vi "Motor Status Wait Z.vi"(2 "Error In":errorcluster, 3 "Reference In":refnum<class "_Controller.lvclass">) -> (0 "Error Out":errorcluster, 1 "Reference Out":refnum<class "_Controller.lvclass">)   [LabVIEW 2020]
doc: "Waits for motor Z to be in idle (i.e. not moving). This is done to ensure motor Z has completed any neccessary movement before sending the next command. Otherwise a pulsing error is obtained.\n\nArgs:\n\nReference In: Incoming communication (reference) between LabView and the scanning rig controller\nError In: Checks for any errors with the incoming communication (reference)\n\nReturns:\n\nReference Out: Output communnication (reference) between LabView and controller\nError Out: Checks for any error with output communication (reference)"
uses:
  <instrlib>/Arcus Ethernet Driver 1.0.0/ArcusEthernetComm/classes/Controller/_Controller.lvclass
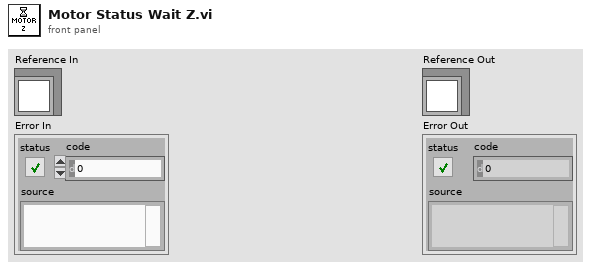
[diagram p1: front panel]
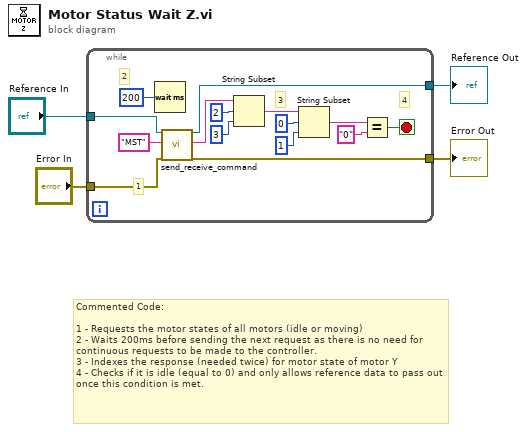
[diagram p0: block diagram]
diagram:
  # "Commented Code:\n\n1 - Requests the motor states of all motors (idle or moving)\n2 - Waits 200ms before sending the next request as there is no need for continuous requests to be made to the controller. \n3 - Indexes the response (needed twice) for motor state of motor Y\n4 - Checks if it is idle (equal to 0) and only allows reference data to pass out once this condition is met."
  n1 = while {
    tunnel: "Reference In" -> [w14]
    tunnel: "Error In" -> [w13]
    tunnel: [w10] -> w2
    tunnel: [w9] -> w1
    stop <- w11 stop-if-true
    # "4"
    # "3"
    # "2"
    # "1"
    n2 = Wait (ms)(milliseconds to wait=u32 200) -> ()  [unwired: 1 out]
    n3 = call <instrlib>:"send_receive_command.vi"("reference (in)"=w14, "ASCII Command (in)"="MST", "error in (no error)"=w13) -> ("reference (out)"=w10:refnum<class "_Controller.lvclass">, "response (out)"=w15:string, "error out"=w9:errorcluster)  [unwired: 12 in, 2 out]
    n4 = String Subset(string=w15, offset (0)=2, length (rest)=3 ("length (rest)")) -> (substring=w8:string)
    n5 = String Subset(string=w8, offset (0)=0, length (rest)=1 ("length (rest)")) -> (substring=w5:string)
    n6 = Equal?(x=w5, y="0") -> (x = y?=w11:bool)
  }
  "Reference Out" <- w2
  "Error Out" <- w1
